vi "SCOPE.vi"() -> ()   [LabVIEW 2013]
doc: "Example: Quick Start\n\nRecommended Input Signal: 2V pk-pk @ 1kHz\n\nDevices Supported: Refer to NI Example Finder\n\nLabVIEW Description:\n\nThis example configures all the oscilloscope's vertical, horizontal, and triggering properties before every acquisition. It allows you to experiment with numerous configurations.\n\nThe niScope Probe Compensation signal is enabled, and is enabled so that it can be used as a signal source, when connected to an acquistion channel. This VI starts the 1 kHz square wave output on PFI 1, which is typically used for probe compensation.\n\nAfter the Read VI is called to acquire a waveform, the Fetch Measurement Stats VI is used to perform the desired scalar measurement analysis on the waveform. NI-SCOPE keeps a history of each measurement's results, which allows it to retrieve the statistics computed over multiple acquisitions. These statistics include the mean, standard deviation, min, max and number of acquisitions used in the statistics. The statistics are updated once per acquisition when the measurement is fetched. \n\n\nKeep in mind that not all oscilloscopes support all the features in this example. The NI High Speed Digitizers Help includes a table of supported features for each device."
uses:
  <instrlib>/niScope/Controls/niScope scalar measurement.ctl
  <instrlib>/niScope/Configure/Trigger/niScope Configure Trigger Edge.vi
  <instrlib>/niScope/Acquire/niScope Multi Read Cluster.vi
  <instrlib>/niScope/Measurements/niScope Fetch Measurement.vi
panel:
  in  "scalar measurement":T1=4000 caption="Scalar Measurement" items=["None"=4000, "Frequency"=2, "Average Frequency"=1016, "FFT Frequency"=1008, "Period"=3, "Average Period"=1015, "Rise Time"=0, "Fall Time"=1, "Rising Slew Rate"=1010, "Falling Slew Rate"=1011, "Overshoot"=18, "Preshoot"=19, "Voltage RMS"=4, "Voltage Cycle RMS"=16, "AC Estimate"=1012, "FFT Amplitude"=1009, "Voltage Average"=10, "Voltage Cycle Average"=17, "DC Estimate"=1013, "Voltage Max"=6, "Voltage Min"=7, "Voltage Peak-to-Peak"=5, "Voltage High"=8, "Voltage Low"=9, "Voltage Amplitude"=15, "Voltage Top"=1007, "Voltage Base"=1006, "Voltage Base-to-Top"=1017, "Negative Width"=11, "Positive Width"=12, "Negative Duty Cycle"=13, "Positive Duty Cycle"=14, "Integral"=1005, "Area"=1003, "Cycle Area"=1004, "Time Delay"=1014, "Phase Delay"=1018, "Low Ref Volts"=1000, "Mid Ref Volts"=1001, "High Ref Volts"=1002, "Volt. Hist. Mean"=2000, "Volt. Hist. Stdev"=2001, "Volt. Hist. Median"=2003, "Volt. Hist. Mode"=2010, "Volt. Hist. Max"=2005, "Volt. Hist. Min"=2006, "Volt. Hist. Peak-to-Peak"=2002, "Volt. Hist. Mean + Stdev"=2007, "Volt. Hist. Mean + 2 Stdev"=2008, "Volt. Hist. Mean + 3 Stdev"=2009, "Volt. Hist. Hits"=2004, "Volt. Hist. New Hits"=2011, "Time Hist. Mean"=3000, "Time Hist. Stdev"=3001, "Time Hist. Median"=3003, "Time Hist. Mode"=3010, "Time Hist. Max"=3005, "Time Hist. Min"=3006, "Time Hist. Peak-to-Peak"=3002, "Time Hist. Mean + Stdev"=3007, "Time Hist. Mean + 2 Stdev"=3008, "Time Hist. Mean + 3 Stdev"=3009, "Time Hist. Hits"=3004, "Time Hist. New Hits"=3011]
  out "scalar result":dbl caption="Scalar Result"
  in  "Input Impedance":u32(ring) items=["1 mega ohm"=0, "50 ohms"=2]
  in  "Trigger Modifier":i32(ring)=2 items=["None"=1, "Auto Trigger"=2]
  in  "Coupling":u16(ring)=1 items=["AC"=0, "DC"=1, "HF Reject"=3, "LF Reject"=4, "AC Plus HF Reject"=1001]
  in  "Trigger Slope":i32(ring) items=["Positive", "Negative"]
  in  "Trigger Level (V)":dbl=0.5 caption="Trigger Level" format="%.2f"
  in  "Vertical Coupling":i32(ring)=1 items=["AC", "DC", "Ground"]
  in  "Min. Sample Rate":dbl=10000000.0 format="%#_6p"
  in  "Vertical Range (V)":dbl=5.0 format="%_3g"
  in  "Min Record Length":i32=40000
  out "Waveform From Scope":T2(graph) caption="Waveform from Scope"
  in  "Channel(s)":string="0" caption="Channel"
  in  "Resource Name":refnum<k15>="DAQ::1"
  # "Overview: This example features a faster getting started experience.\nRequirements: NI-SCOPE\nInstructions:\n1.  Select a valid NI-SCOPE resource.\n2. Connect an input signal to Channel 0, it should be a square wave, 2V pk-pk @ 1kHz.\n     Note: On supported digitizers, a signal is generated on PFI 1 if needed for signal input.\n3.  Run the VI."
  # "Vertical"
  # "Horizontal"
  # "Triggering"
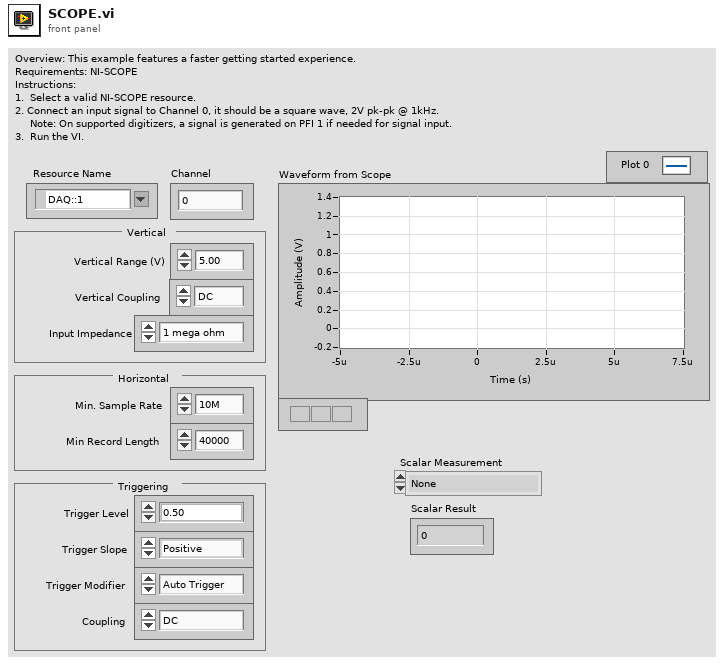
[diagram p1: front panel]
types:
  T1 = typedef "niScope scalar measurement.ctl" = i32
  T2 = cluster{"relativeInitialX":dbl, "xIncrement":dbl, "wfm":dbl[]}[]
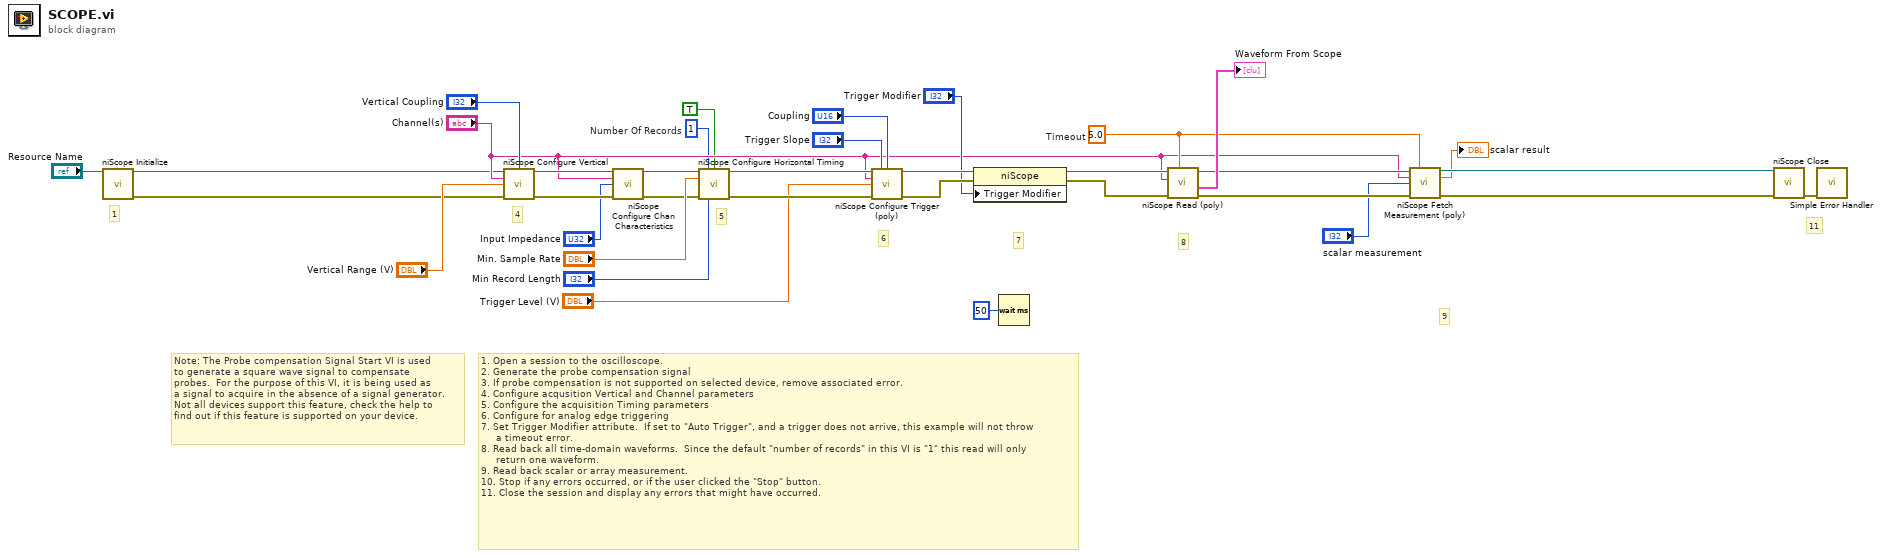
[diagram p0: block diagram]
diagram:
  w6 = 1  # Number Of Records
  w13 = 5.0  # Timeout
  # "9"
  # "8"
  # "6"
  # "5"
  # "4"
  # "7"
  # "Note: The Probe compensation Signal Start VI is used\nto generate a square wave signal to compensate\nprobes.  For the purpose of this VI, it is being used as\na signal to acquire in the absence of a signal generator.\nNot all devices support this feature, check the help to\nfind out if this feature is supported on your device."
  # "11"
  # "1"
  # "1. Open a session to the oscilloscope.\n2. Generate the probe compensation signal \n3. If probe compensation is not supported on selected device, remove associated error.\n4. Configure acqusition Vertical and Channel parameters\n5. Configure the acquisition Timing parameters\n6. Configure for analog edge triggering\n7. Set Trigger Modifier attribute.  If set to \"Auto Trigger\", and a trigger does not arrive, this example will not throw\n     a timeout error.\n8. Read back all time-domain waveforms.  Since the default \"number of records\" in this VI is \"1\" this read will only\n     return one waveform.\n9. Read back scalar or array measurement.\n10. Stop if any errors occurred, or if the user clicked the \"Stop\" button.\n11. Close the session and display any errors that might have occurred."
  n1 = call <instrlib>:"niScope Initialize.vi"("resource name"="Resource Name") -> ("instrument handle"=w3:refnum<k15>, "error out"=w4:errorcluster)  [unwired: 13 in]
  n2 = call <instrlib>:"niScope Configure Vertical.vi"("instrument handle"=w3, "vertical coupling"="Vertical Coupling", "channels"="Channel(s)", "vertical range"="Vertical Range (V)", "error in"=w4) -> ("instrument handle out"=w11:refnum<k15>, "error out"=w12:errorcluster)  [unwired: 9 in]
  n3 = call <instrlib>:"niScope Configure Chan Characteristics.vi"("instrument handle"=w11, "channels"="Channel(s)", "input impedance"="Input Impedance", "error in"=w12) -> ("instrument handle out"=w9:refnum<k15>, "error out"=w8:errorcluster)  [unwired: 10 in]
  n4 = call <instrlib>:"niScope Configure Horizontal Timing.vi"("instrument handle"=w9, "number of records"=w6, "enforce realtime"=TRUE ("Enforce Realtime"), "min sample rate"="Min. Sample Rate", "error in"=w8, "min record length"="Min Record Length") -> ("instrument handle out"=w25:refnum<k15>, "error out"=w26:errorcluster)  [unwired: 8 in]
  n5 = call-poly <instrlib>:"niScope Configure Trigger (poly).vi"("instrument handle"=w25, "trigger slope"="Trigger Slope", "trigger coupling"="Coupling", "trigger source"="Channel(s)", "trigger level"="Trigger Level (V)", "error in"=w26) -> ("instrument handle out"=w18:refnum<k15>, "error out"=w17:errorcluster)  [unwired: 8 in]
  n6 = property class="niScope"(reference=w18, error in=w17, "Trigger Modifier"="Trigger Modifier") -> (reference out=w14:refnum<k15>, error out=w15:errorcluster)
  n7 = Wait (ms)(milliseconds to wait=u32 50 ("Millisecond Multiple")) -> ()  [unwired: 1 out]
  n8 = call-poly <instrlib>:"niScope Read (poly).vi"("timeout"=w13, "error in"=w15, "channels"="Channel(s)", "instrument handle"=w14) -> ("error out"=w22:errorcluster, "waveform"=→"Waveform From Scope":T2, "instrument handle out"=w23:refnum<k15>)  [unwired: 4 in, 1 out]
  n9 = call-poly <instrlib>:"niScope Fetch Measurement (poly).vi"("instrument handle"=w23, "timeout"=w13, "channels"="Channel(s)", "scalar measurement"="scalar measurement", "error in"=w22) -> ("instrument handle out"=w33:refnum<k15>, "result"=→"scalar result":dbl, "error out"=w32:errorcluster)  [unwired: 8 in]
  n10 = call <instrlib>:"niScope Close.vi"("instrument handle"=w33, "error in"=w32) -> ("error out"=w34:errorcluster)  [unwired: 13 in]
  n11 = call <vilib>:"Simple Error Handler.vi"("error in (no error)"=w34) -> ()  [unwired: 4 in, 5 out]
